vi "Actor Core.vi"(8 "error in":errorcluster, 11 "Appearance Actor in":refnum<class "Appearance Actor.lvclass">) -> (0 "error out":errorcluster, 3 "Actor out":refnum<class "Actor.lvclass">)   [LabVIEW 2021, in "Appearance Actor.lvlib" / "Appearance Actor.lvclass"]
doc: "The user interface for this panel.\n\n----\nPlease see the following web address for additional documentation and tutorial information:\nhttp://www.mooregoodideas.com/mgi-panel-manager/\n\nAuthor: Derek Trepanier\n\nCopyright (c) 2018, Moore Good Ideas, Inc.\n\nAll rights reserved.\n\nRedistribution and use in source and binary forms, with or without modification, are permitted provided that the following conditions are met:\n\n * Redistributions of source code must retain the above copyright notice, this list of conditions and the following disclaimer.\n * Redistributions in binary form must reproduce the above copyright notice, this list of conditions and the following disclaimer in the documentation and/or other materials provided with the distribution.\n * Neither the name of Moore Good Ideas, Inc. nor the names of its contributors may be used to endorse or promote products derived from this software without specific prior written permission.\n\nTHIS SOFTWARE IS PROVIDED BY THE COPYRIGHT HOLDERS AND CONTRIBUTORS \"AS IS\" AND ANY EXPRESS OR IMPLIED WARRANTIES, INCLUDING, BUT NOT LIMITED TO, THE IMPLIED WARRANTIES OF MERCHANTABILITY AND FITNESS FOR A PARTICULAR PURPOSE ARE DISCLAIMED. IN NO EVENT SHALL THE COPYRIGHT OWNER OR CONTRIBUTORS BE LIABLE FOR ANY DIRECT, INDIRECT, INCIDENTAL, SPECIAL, EXEMPLARY, OR CONSEQUENTIAL DAMAGES (INCLUDING, BUT NOT LIMITED TO, PROCUREMENT OF SUBSTITUTE GOODS OR SERVICES; LOSS OF USE, DATA, OR PROFITS; OR BUSINESS INTERRUPTION) HOWEVER CAUSED AND ON ANY THEORY OF LIABILITY, WHETHER IN CONTRACT, STRICT LIABILITY, OR TORT (INCLUDING NEGLIGENCE OR OTHERWISE) ARISING IN ANY WAY OUT OF THE USE OF THIS SOFTWARE, EVEN IF ADVISED OF THE POSSIBILITY OF SUCH DAMAGE."
uses:
  Appearance Actor.lvclass
  <vilib>/ActorFramework/Actor/Actor.lvclass
  Appearance Actor.lvclass/Appearance Actor.ctl
  <userlib>/_MGI/Application Control/MGI VI Reference/MGI Caller's VI Reference.vi
  <vilib>/MGI/Panel Manager/Panel Actor/Panel Actor/Panel Actor.lvclass
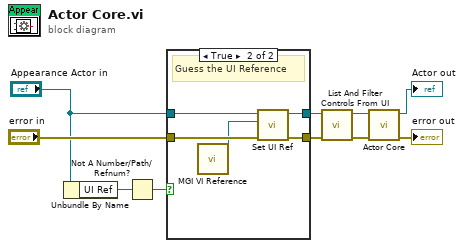
[diagram p0: block diagram]
diagram:
  n1 = Unbundle By Name("Appearance Actor in") -> ("UI Ref"=w6:refnum<vi>)
  n2 = Not A Number/Path/Refnum?(number/path/refnum=w6) -> (NaN/Path/Refnum?=w2:bool)
  n3 = case shown="True" w2 {
    tunnel: "error in" -> [w11 w17]
    tunnel: [w11 w16] -> w5
    tunnel: [w12 w15] -> w4
    tunnel: "Appearance Actor in" -> [w12 w14]
    frame False {
      # "UI Reference Valid"
    }
    frame True {
      # "Guess the UI Reference"
      n4 = call-poly <userlib>:"MGI VI Reference.vi"() -> ("Caller's VI Reference"=w13:refnum<vi>)  [unwired: 1 in]
      n5 = call "Set UI Ref.vi"("error in (no error)"=w17, "UI Ref"=w13, "Appearance Actor in"=w14) -> ("error out"=w16:errorcluster, "Appearance Actor out"=w15:refnum<class "Appearance Actor.lvclass">)  [unwired: 7 in]
    }
  }
  n6 = call "List And Filter Controls From UI.vi"("Error In"=w5, "Appearance Actor In"=w4) -> ("Error Out"=w1:errorcluster, "Appearance Actor Out"=w7:refnum<class "Appearance Actor.lvclass">)  [unwired: 8 in]
  n7 = call-parent "Actor Core.vi"("error in"=w1, "Panel Actor in"=w7) -> ("error out"=→"error out":errorcluster, "Actor out"=→"Actor out":refnum<class "Actor.lvclass">)  [unwired: 8 in]
